vi "dfd_Get Lattice Type Id.vi"(0 "structure type":T3) -> (1 "lattice type":T2, 2 "section type":T1(ring))   [LabVIEW 2017, in "NI_DigFilterLicensed.lvlib"]
uses:
  <vilib>/addons/Digital Filter Design/NI_DigFilterLicensed.lvlib
  <vilib>/addons/Digital Filter Design/_Objects.llb/DFD Filter Structure Type Selector.ctl
  <vilib>/addons/Digital Filter Design/_Objects.llb/DFD Lattice Type.ctl
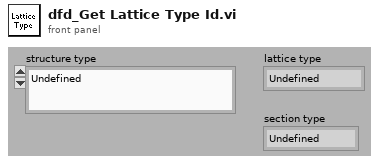
[diagram p1: front panel]
types:
  T1 = enum16{"Undefined", "Basic", "One Multiplier", "Normalized"}
  T2 = typedef "NI_DigFilterLicensed.lvlib/DFD Lattice Type.ctl" = enum16{"Undefined", "Lattice Allpass", "Lattice AR", "Lattice MA (min)", "Lattice MA (max)", "Lattice ARMA"}
  T3 = typedef "NI_DigFilterLicensed.lvlib/DFD Filter Structure Type Selector.ctl" = enum16{"Undefined", "FIR Direct Form", "FIR Direct Form Transposed", "FIR Symmetric", "FIR Antisymmetric", "IIR Direct Form I", "IIR Direct Form I Transposed", "IIR Direct Form II", "IIR Direct Form II Transposed", "IIR Cascaded Second Order Sections Form I", "IIR Cascaded Second Order Sections Form I Transposed", "IIR Cascaded Second Order Sections Form II", "IIR Cascaded Second Order Sections Form II Transposed", "Lattice Allpass (basic sections)", "Lattice Allpass (one multiplier sections)", "Lattice Allpass (normalized sections)", "Lattice AR (basic sections)", "Lattice AR (one multiplier sections)", "Lattice AR (normalized sections)", "Lattice MA (minimum phase)", "Lattice MA (maximum phase)", "Lattice ARMA (basic sections)", "Lattice ARMA (one multiplier sections)", "Lattice ARMA (normalized sections)"}
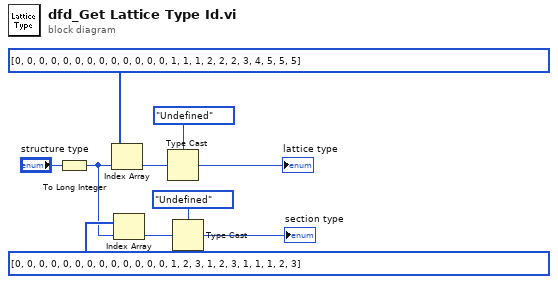
[diagram p0: block diagram]
diagram:
  n1 = To Long Integer(number="structure type") -> (32bit integer=w4:i32)
  n2 = Index Array(array=u16[] [0, 0, 0, 0, 0, 0, 0, 0, 0, 0, 0, 0, 0, 1, 1, 1, 2, 2, 2, 3, 4, 5, 5, 5], index=w4) -> (element=w9:u16)
  n3 = Index Array(array=u16[] [0, 0, 0, 0, 0, 0, 0, 0, 0, 0, 0, 0, 0, 1, 2, 3, 1, 2, 3, 1, 1, 1, 2, 3], index=w4) -> (element=w3:u16)
  n4 = Type Cast(type=DFD_Lattice_Type."Undefined" ("lattice type"), x=w9) -> (*(type *) &x=→"lattice type":T2)
  n5 = Type Cast(type=T1."Undefined" ("section type"), x=w3) -> (*(type *) &x=→"section type":T1)
